vi "Robot Global Data.vi"() -> ()   [LabVIEW 2016]
doc: "This global VI can contain as many global variables as you need. Place a control on the panel, give it a good name. To read or write to it from a VI, drag the icon to the diagram of that VI. You can also drag from the project. Click on the node to change which global you access. You shouldn't have multiple locations writing to a global or it will cause a race-condition."
uses:
  <vilib>/Rock Robotics/WPI/Camera/WPI_CameraImageSize.ctl
  <vilib>/Rock Robotics/WPI/DriverStation/WPI_DriverStationRobotMode2.ctl
panel:
  in  "Turning off":bool
  in  "First shoot loop":bool
  in  "Close to peg":bool
  in  "Feeder Speed":dbl=0.9
  in  "Shoot Wheel RPM":dbl
  in  "Run Shoot Wheel":bool
  in  "Ball In Shooter":bool
  in  "Climbing?":bool
  in  "Invert Climb":bool
  in  "Gear Grab Closed":bool
  in  "Gear Up":bool
  in  "Lift Toggle":bool
  in  "Shoot Toggle":bool
  in  "Enable Interval Thump":bool
  in  "Thumper Interval":bool
  in  "NumValuesInTable":dbl=88.0
  in  "Gear Grab Release":bool
  in  "Gear Lift Stat":bool
  in  "Gear Box Stat":bool
  in  "Shoot Latch":bool
  in  "Temp Shoot Speed":dbl=0.7083133333333334
  in  "Gear plate pressed?":bool
  in  "Current RPM":dbl=1.0
  in  "Gear In":bool
  in  "Man Gear Latch":bool
  in  "Pixy In Use":bool
  in  "Gear Ready":bool
  in  "Teleop Elapsed":dbl=112.209
  in  "Blink":bool
  in  "Warning":bool
  in  "Estop":bool
  in  "RPM 4":dbl=0.85
  in  "RPM 3":dbl=0.95
  in  "RPM 2":dbl=0.9
  in  "RPM 1":dbl=1.0
  in  "RPM Shift":dbl
  in  "Climb Speed":dbl=1.0
  in  "Object Width":dbl=23.333333333333332
  in  "Gear In Delay":dbl=0.2
  in  "Fast Drive":dbl=100.0
  in  "Slow Drive":dbl=50.0
  in  "Object X":dbl=-7.666666666666667
  in  "Object":bool
  in  "Object Height":dbl=19.0
  in  "Pixy Output":dbl=-7.666666666666667
  in  "Sonar Distance":dbl
  in  "Shoot Encoder":dbl
  in  "Robot Mode":T1=enum."Finish"
  in  "image size":T2=enum."320x240"
  in  "Enable Vision":bool
  # "Misc. Variables"
  # "Photon Notification System"
  # "Pixy Vision Processing Variables"
  # "Gear Placement Variables"
  # "Note: Other Variables\nare located in\nPeriodic Tasks"
  # "Passive System"
  # "Used In Periodic"
  # "Shooting Variables"
  # "Note: Other Variables\nare located in\nPeriodic Tasks"
  # "Automated Aiming"
  # "Active System"
  # "Unused"
  # "Drivetrain Variables"
  # "Climbing"
  # "Note: Turn Impementaion\nwas here until a failure\nof another system caused\na rollback. An example is \nin Disabled case of \nDriveControllerBuffer vi"
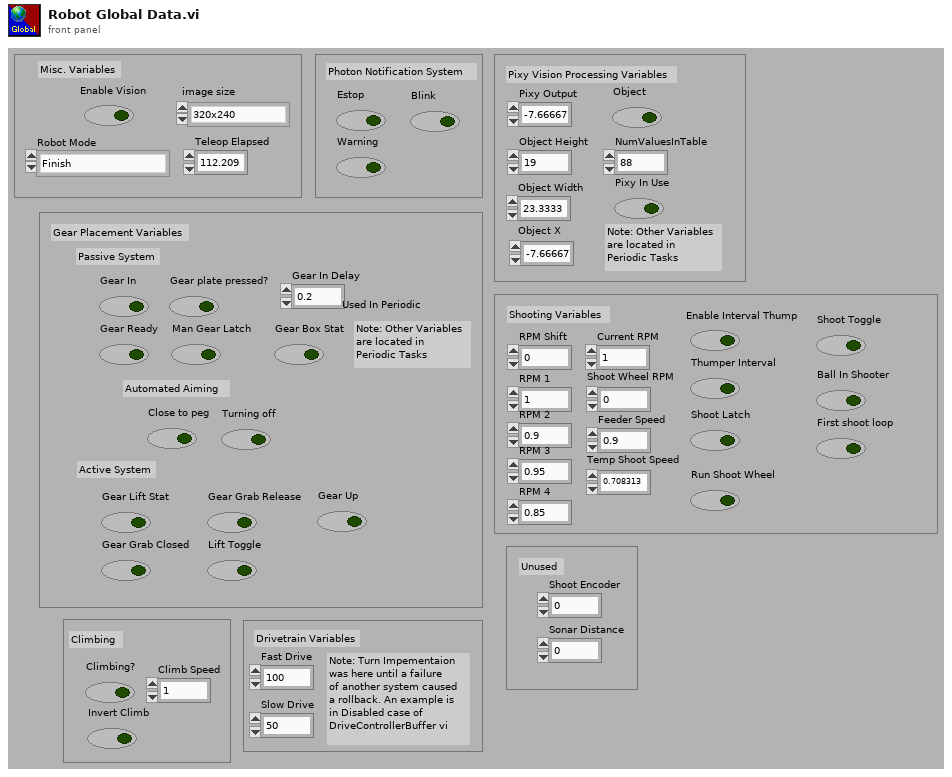
[diagram p1: front panel]
types:
  T1 = typedef "WPI_DriverStationRobotMode2.ctl" = enum16{"Autonomous Disabled", "Autonomous Enabled", "Teleop Disabled", "Teleop Enabled", "Disconnected", "Finish", "Test Disabled", "Test Enabled", "Emergency Stopped"}
  T2 = typedef "WPI_CameraImageSize.ctl" = enum16{"640x480", "320x240", "160x120", "Custom"}
diagram:
